vi "Read SkillRef.vi"(8 "error in (no error)":errorcluster, 11 "SkillStateMachine in":refnum<class "SkillStateMachine.lvclass">) -> (0 "error out":errorcluster, 2 "SkillRef":refnum<class "Skill.lvclass">[](array[class]), 3 "SkillStateMachine out":refnum<class "SkillStateMachine.lvclass">)   [LabVIEW 2018, in "SkillStateMachine.lvclass"]
uses:
  SkillStateMachine.lvclass
  Skill_class/Skill.lvclass
  SkillStateMachine.lvclass/SkillStateMachine.ctl
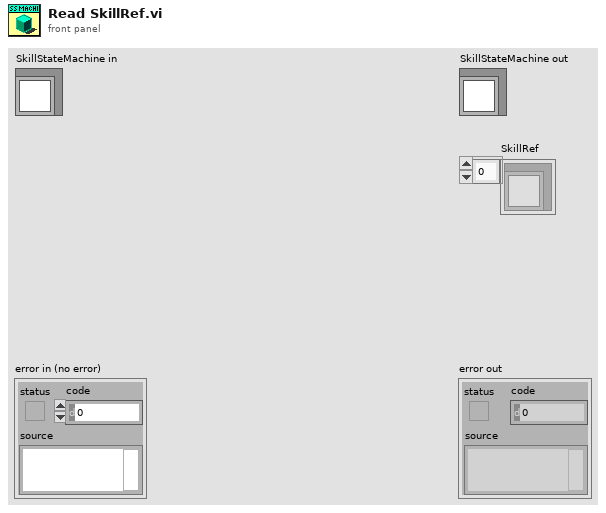
[diagram p1: front panel]
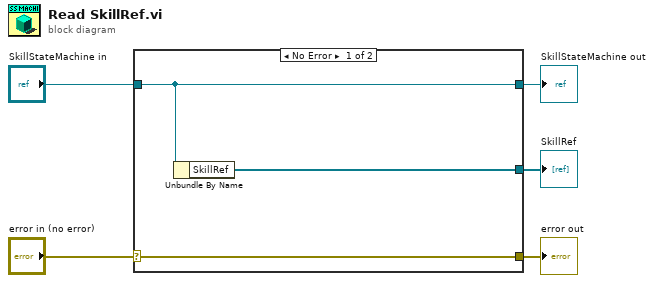
[diagram p0: block diagram]
diagram:
  n1 = case shown="No Error" "error in (no error)" {
    selector: "error in (no error)" -> [w8 w9]
    tunnel: [w8 w9] -> w4
    tunnel: [w7 w10] -> w2
    tunnel: "SkillStateMachine in" -> [w7 w10]
    tunnel: [w6 _] -> w1
    frame No Error {
      n2 = Unbundle By Name(w7) -> ("SkillRef"=w6:refnum<class "Skill.lvclass">[])
    }
    frame Error {
    }
  }
  "error out" <- w4
  "SkillStateMachine out" <- w2
  "SkillRef" <- w1
